vi "MainFlush.vi"(8 "Error":errorcluster) -> (0 "Error Out":errorcluster, 3 "Elements In Queue Out":T1[](array[typedef]))   [LabVIEW 2022 SP3]
doc: "The function removes all the elements in the Queue and returns them."
uses:
  Type Def/MainStates Cluster.ctl
  Type Def/MainStates.ctl
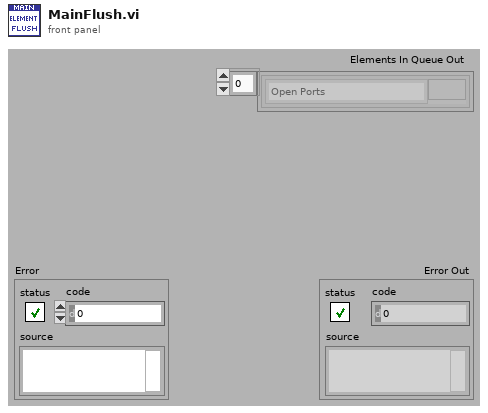
[diagram p1: front panel]
types:
  T1 = typedef "MainStates Cluster.ctl" = cluster{"States":T2, "Data":variant}
  T2 = typedef "MainStates.ctl" = enum16{"Open Ports", "Close Ports", "Main", "Settings", "Voltaje", "Probe", "Lenguaje", "Callibration", "Exit", "Voltage Test", "Test 2", "End test"}
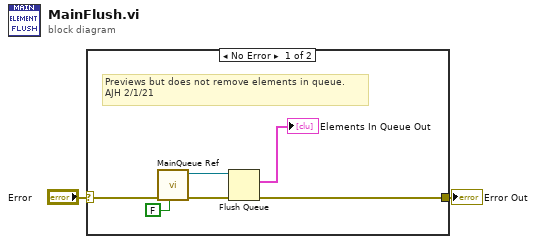
[diagram p0: block diagram]
diagram:
  n1 = case shown="No Error" "Error" {
    selector: "Error" -> [w7 w9]
    tunnel: [w3 w9] -> w1
    frame No Error {
      # "Previews but does not remove elements in queue.\nAJH 2/1/21"
      n2 = call "MainQueue Ref.vi"("Write:T/Read:(F)"=FALSE ("Write:T/Read:F"), "error in"=w7) -> ("error out"=w5:errorcluster, "queue out"=w6:refnum<queue>)  [unwired: 8 in]
      n3 = Flush Queue(queue=w6, error in (no error)=w5) -> (remaining elements=→"Elements In Queue Out":T1[], error out=w3:errorcluster)  [unwired: 1 out]
    }
    frame Error {
    }
  }
  "Error Out" <- w1
